vi "Get Cluster Element Names.vi"(8 "error in (no error)":errorcluster, 11 "Cluster in":variant) -> (0 "error out":errorcluster, 2 "Names":string[](array[string]), 3 "Cluster  out":variant)   [LabVIEW 2015, in "Scripting.lvlib"]
uses:
  Scripting.lvlib
  <vilib>/Utility/Data Type/NI_Data Type.lvlib
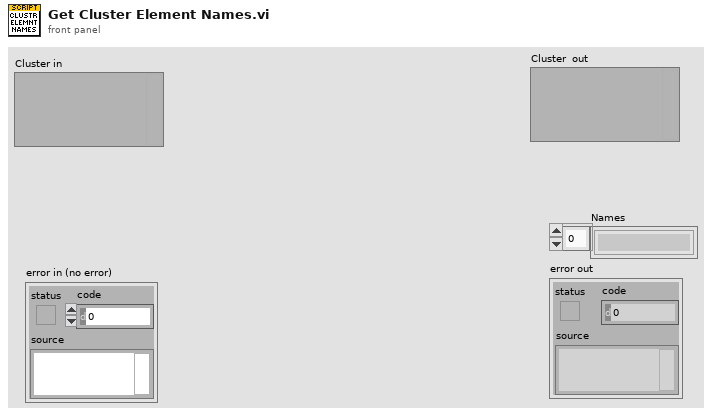
[diagram p1: front panel]
types:
  T1 = typedef "NI_Data Type.lvlib/Data Type.ctl" = enum8{"Invalid Type", "Void", "I8", "I16", "I32", "I64", "U8", "U16", "U32", "U64", "Single Float", "Double Float", "Extended Float", "Single Complex", "Double Complex", "Extended Complex", "Enum U8", "Enum U16", "Enum U32", "Enum U64", "Single Float With Unit", "Double Float With Unit", "Extended Float With Unit", "Single Complex with Unit", "Double Complex with Unit", "Extended Complex with Unit", "Boolean", "String", "Path", "Picture", "Tag", "Array", "Cluster", "Variant", "LV Variant", "Waveform", "Timestamp", "Digital Waveform", "Digital Data", "ExpressData", "Refnum", "External Data", "VI", "Poly VI", "LabVIEW Class Instance", "Fixed Point"}
  T2 = cluster{"Array Element Data Type":variant, string}
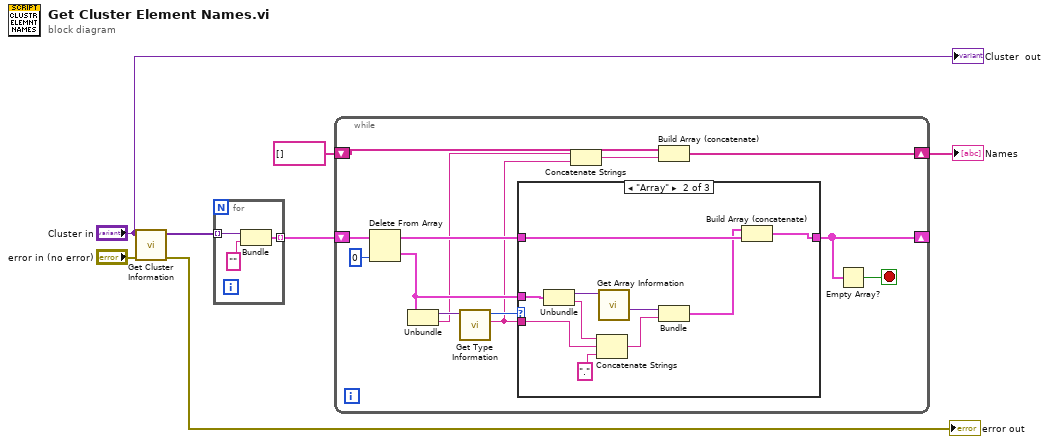
[diagram p0: block diagram]
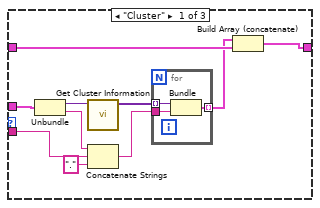
[diagram p2: hidden frame]
diagram:
  n1 = call <vilib>:"Get Cluster Information.vi"("error in (no error)"="error in (no error)", "Variant"="Cluster in") -> ("error out"=→"error out":errorcluster, "Cluster Elements"=w4:variant[])  [unwired: 8 in]
  n2 = for {
    tunnel: w4 -> [w10] mode=indexing
    tunnel: [w9] -> w3 mode=indexing
    n3 = Bundle("Variant"=w10, "Name"="") -> (w9:cluster{"Variant":variant, "Name":string})  [unwired: 1 in]
  }
  n4 = while {
    shift-right: [w19] -> w5
    shift-left: string[] [] -> [w13]
    shift-right: [w12] -> _
    shift-left: w3 -> [w23]
    stop <- w18 stop-if-true
    n5 = Delete From Array(array=w23, index=0) -> (deleted portion=w17:cluster{"Variant":variant, "Name":string}, array with subset deleted=w21:cluster{"Variant":variant, "Name":string}[])  [unwired: 1 in]
    n6 = Unbundle(w17) -> ("Variant"=w16:variant, "Name"=w14:string)
    n7 = call <vilib>:"Get Type Information.vi"("Variant"=w16) -> ("Name"=w11:string, "Type"=w22:T1)  [unwired: 6 in, 3 out]
    n8 = case shown="\"Array\"" w22 {
      tunnel: w21 -> [w33 w46 w47]
      tunnel: [w28 w44 w47] -> w12
      tunnel: w17 -> [w27 w43 _]
      tunnel: w11 -> [w24 w37 _]
      frame "Cluster" {
        n9 = Unbundle(w27) -> ("Variant"=w26:variant, "Name"=w25:string)
        n10 = call <vilib>:"Get Cluster Information.vi"("Variant"=w26) -> ("Cluster Elements"=w31:variant[])  [unwired: 9 in, 1 out]
        n11 = Concatenate Strings(w25, w24, "." ("string")) -> (w30:string)
        n12 = for {
          tunnel: w31 -> [w36] mode=indexing
          tunnel: w30 -> [w35]
          tunnel: [w34] -> w29 mode=indexing
          n13 = Bundle("Variant"=w36, w35) -> (w34:cluster{"Variant":variant, string})  [unwired: 1 in]
        }
        n14 = Build Array (concatenate)(w29, w33) -> (w28:cluster{"Variant":variant, "Name":string}[])
      }
      frame "Array" {
        n15 = Unbundle(w43) -> ("Variant"=w42:variant, "Name"=w38:string)
        n16 = Concatenate Strings(w38, w37, "." ("string")) -> (w40:string)
        n17 = call <vilib>:"Get Array Information.vi"("Variant"=w42) -> ("Array Element Data Type"=w41:variant)  [unwired: 7 in, 3 out]
        n18 = Bundle("Array Element Data Type"=w41, w40) -> (w39:T2)  [unwired: 1 in]
        n19 = Build Array (concatenate)(w39, w46) -> (w44:cluster{"Variant":variant, "Name":string}[])
      }
      frame Default {
      }
    }
    n20 = Concatenate Strings(w14, w11) -> (w15:string)
    n21 = Build Array (concatenate)(w13, w15) -> (w19:string[])
    n22 = Empty Array?(array=w12) -> (empty?=w18:bool)
  }
  "Names" <- w5
  "Cluster  out" <- "Cluster in"
